vi "ROS_Publish.vi"() -> ()   [LabVIEW 2020]
uses:
  C:/Users/NI/Desktop/ROS/Release/ROSPublisherClass.dll
  Release/ROSPublisherClass.dll
panel:
  out "Numeric 2":i32
  out "Time 2":u32
  out "Time Array 2":u32[](array[numeric])
  out "Time Array":u32[](array[numeric])
  out "Time":u32
  out "Numeric":i32
  out "error out":errorcluster
  in  "stop":bool
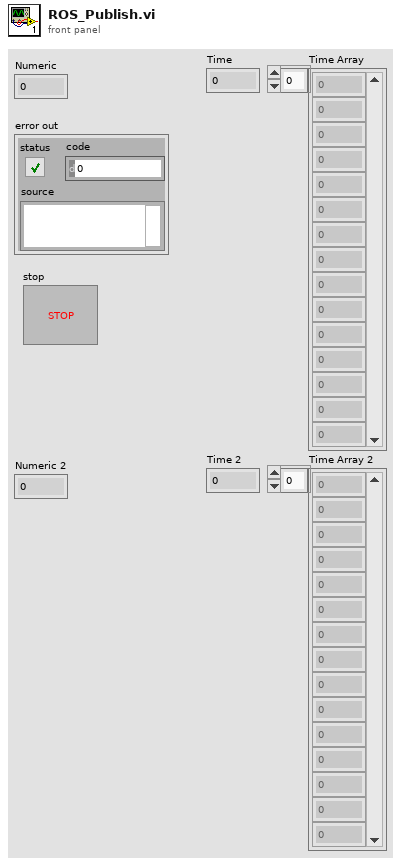
[diagram p1: front panel]
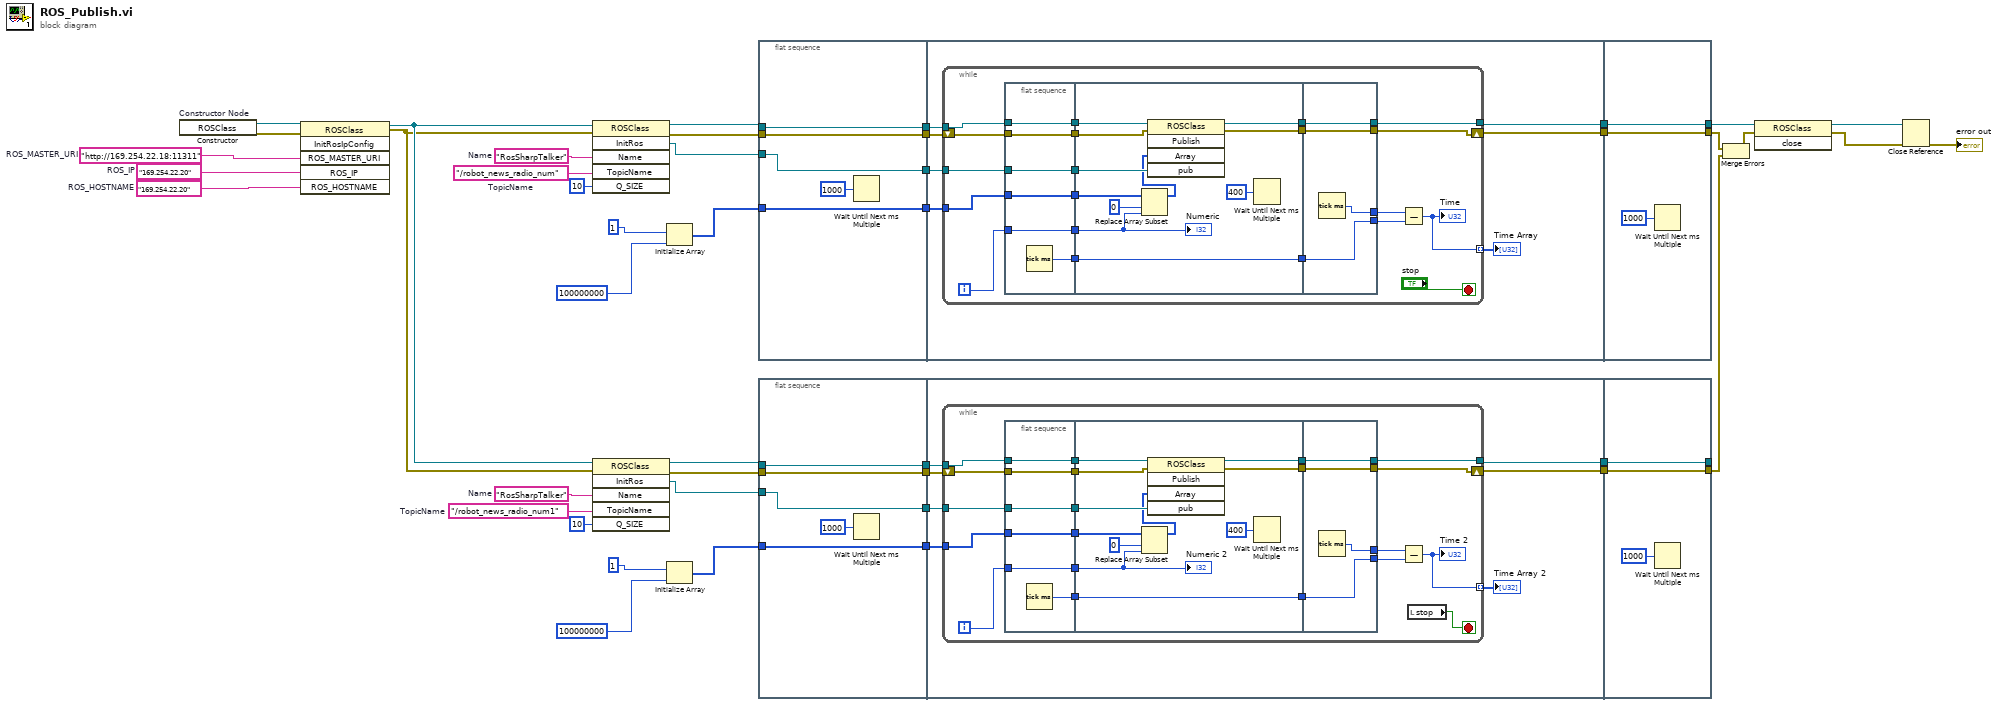
[diagram p0: block diagram]
diagram:
  w13 = "/robot_news_radio_num1"  # TopicName
  w12 = "RosSharpTalker"  # Name
  w22 = "/robot_news_radio_num"  # TopicName
  w23 = "RosSharpTalker"  # Name
  w24 = "169.254.22.20"  # ROS_HOSTNAME
  w26 = "http://169.254.22.18:11311"  # ROS_MASTER_URI
  w25 = "169.254.22.20"  # ROS_IP
  n1 = constructor on="Constructor Node" class="ROSClass"() -> (reference out=w41:refnum<k24>, error out=w30:errorcluster)  [unwired: 3 in, 1 out]
  n2 = invoke class="ROSClass" method="InitRosIpConfig"(reference=w41, error in=w30, "ROS_MASTER_URI"=w26, "ROS_IP"=w25, "ROS_HOSTNAME"=w24) -> (reference out=w5:refnum<k24>, error out=w4:errorcluster)  [unwired: 1 in, 4 out]
  n3 = invoke class="ROSClass" method="InitRos"(reference=w5, error in=w4, "Name"=w23, "TopicName"=w22, "Q_SIZE"=10) -> (reference out=w28:refnum<k24>, error out=w29:errorcluster, "InitRos"=w27:refnum<k24>)  [unwired: 1 in, 3 out]
  n4 = invoke class="ROSClass" method="InitRos"(reference=w5, error in=w4, "Name"=w12, "TopicName"=w13, "Q_SIZE"=10) -> (reference out=w10:refnum<k24>, error out=w9:errorcluster, "InitRos"=w11:refnum<k24>)  [unwired: 1 in, 3 out]
  n5 = Initialize Array(u8 1, 100000000 ("dimension size")) -> (w36:u8[])
  n6 = Initialize Array(u8 1, 100000000 ("dimension size")) -> (w8:u8[])
  n7 = flat-sequence {
    tunnel: w29 -> [w48]
    tunnel: w28 -> [w49]
    tunnel: [w49] -> w43
    tunnel: [w48] -> w42
    tunnel: w27 -> [w46]
    tunnel: [w46] -> w40
    tunnel: [w45] -> w37
    tunnel: w36 -> [w45]
    tunnel: w43 -> [w56]
    tunnel: w42 -> [w55]
    tunnel: w40 -> [w52]
    tunnel: w37 -> [w51]
    tunnel: [w54] -> w32
    tunnel: [w53] -> w31
    tunnel: [w99] -> w3
    tunnel: [w100] -> w44
    tunnel: w32 -> [w100]
    tunnel: w31 -> [w99]
    frame #0 {
      n8 = Wait Until Next ms Multiple(millisecond multiple=u32 1000) -> ()  [unwired: 1 out]
    }
    frame #1 {
      n9 = while {
        tunnel: w56 -> [w75]
        tunnel: [w74] -> w54
        shift-right: [w71] -> w53
        shift-left: w55 -> [w72]
        tunnel: w52 -> [w73]
        tunnel: w51 -> [w70]
        tunnel: [w57] -> w50 mode=indexing
        i -> [w69]
        stop <- "stop" stop-if-true
        n10 = flat-sequence {
          tunnel: w69 -> [w78]
          tunnel: w70 -> [w79]
          tunnel: w72 -> [w80]
          tunnel: w73 -> [w81]
          tunnel: w75 -> [w82]
          tunnel: [w82] -> w68
          tunnel: [w81] -> w67
          tunnel: [w80] -> w66
          tunnel: [w79] -> w65
          tunnel: [w78] -> w64
          tunnel: [w77] -> w58
          tunnel: w68 -> [w93]
          tunnel: w67 -> [w91]
          tunnel: w66 -> [w90]
          tunnel: w65 -> [w87]
          tunnel: w64 -> [w86]
          tunnel: [w92] -> w63
          tunnel: [w89] -> w62
          tunnel: [w83] -> w59
          tunnel: w58 -> [w83]
          tunnel: [w96] -> w71
          tunnel: [w97] -> w74
          tunnel: w63 -> [w97]
          tunnel: w62 -> [w96]
          tunnel: [w95] -> w61
          tunnel: [w94] -> w60
          tunnel: w59 -> [w94]
          frame #0 {
            n11 = Tick Count (ms)() -> (millisecond timer value=w77:u32)
          }
          frame #1 {
            n12 = Replace Array Subset(array=w87, new element=w86, index=0) -> (w84:u8[])
            n13 = invoke class="ROSClass" method="Publish"(reference=w93, error in=w90, "Array"=w84, "pub"=w91) -> (reference out=w92:refnum<k24>, error out=w89:errorcluster)  [unwired: 1 in, 3 out]
            n14 = Wait Until Next ms Multiple(millisecond multiple=u32 400) -> ()  [unwired: 1 out]
            "Numeric" <- w86
          }
          frame #2 {
            n15 = Tick Count (ms)() -> (millisecond timer value=w95:u32)
          }
        }
        n16 = Subtract(x=w61, y=w60) -> (x-y=w57:u32)
        "Time" <- w57
      }
      "Time Array" <- w50
    }
    frame #2 {
      n17 = Wait Until Next ms Multiple(millisecond multiple=u32 1000) -> ()  [unwired: 1 out]
    }
  }
  n18 = flat-sequence {
    tunnel: w9 -> [w104]
    tunnel: w10 -> [w105]
    tunnel: [w105] -> w20
    tunnel: [w104] -> w19
    tunnel: w11 -> [w102]
    tunnel: [w102] -> w18
    tunnel: [w101] -> w17
    tunnel: w8 -> [w101]
    tunnel: w20 -> [w112]
    tunnel: w19 -> [w111]
    tunnel: w18 -> [w108]
    tunnel: w17 -> [w107]
    tunnel: [w110] -> w16
    tunnel: [w109] -> w15
    tunnel: [w155] -> w1
    tunnel: [w156] -> _
    tunnel: w16 -> [w156]
    tunnel: w15 -> [w155]
    frame #0 {
      n19 = Wait Until Next ms Multiple(millisecond multiple=u32 1000) -> ()  [unwired: 1 out]
    }
    frame #1 {
      n20 = while {
        tunnel: w112 -> [w132]
        tunnel: [w131] -> w110
        shift-right: [w128] -> w109
        shift-left: w111 -> [w129]
        tunnel: w108 -> [w130]
        tunnel: w107 -> [w127]
        tunnel: [w114] -> w106 mode=indexing
        i -> [w126]
        stop <- w113 stop-if-true
        n21 = flat-sequence {
          tunnel: w126 -> [w134]
          tunnel: w127 -> [w135]
          tunnel: w129 -> [w136]
          tunnel: w130 -> [w137]
          tunnel: w132 -> [w138]
          tunnel: [w138] -> w125
          tunnel: [w137] -> w124
          tunnel: [w136] -> w123
          tunnel: [w135] -> w122
          tunnel: [w134] -> w121
          tunnel: [w133] -> w115
          tunnel: w125 -> [w149]
          tunnel: w124 -> [w147]
          tunnel: w123 -> [w146]
          tunnel: w122 -> [w143]
          tunnel: w121 -> [w142]
          tunnel: [w148] -> w120
          tunnel: [w145] -> w119
          tunnel: [w139] -> w116
          tunnel: w115 -> [w139]
          tunnel: [w152] -> w128
          tunnel: [w153] -> w131
          tunnel: w120 -> [w153]
          tunnel: w119 -> [w152]
          tunnel: [w151] -> w118
          tunnel: [w150] -> w117
          tunnel: w116 -> [w150]
          frame #0 {
            n22 = Tick Count (ms)() -> (millisecond timer value=w133:u32)
          }
          frame #1 {
            n23 = Replace Array Subset(array=w143, new element=w142, index=0) -> (w140:u8[])
            n24 = invoke class="ROSClass" method="Publish"(reference=w149, error in=w146, "Array"=w140, "pub"=w147) -> (reference out=w148:refnum<k24>, error out=w145:errorcluster)  [unwired: 1 in, 3 out]
            n25 = Wait Until Next ms Multiple(millisecond multiple=u32 400) -> ()  [unwired: 1 out]
            "Numeric 2" <- w142
          }
          frame #2 {
            n26 = Tick Count (ms)() -> (millisecond timer value=w151:u32)
          }
        }
        n27 = Subtract(x=w118, y=w117) -> (x-y=w114:u32)
        "Time 2" <- w114
        n28 = local read "stop"() -> (w113:bool)
      }
      "Time Array 2" <- w106
    }
    frame #2 {
      n29 = Wait Until Next ms Multiple(millisecond multiple=u32 1000) -> ()  [unwired: 1 out]
    }
  }
  n30 = Merge Errors(w3, w1) -> (w2:errorcluster)
  n31 = invoke class="ROSClass" method="close"(reference=w44, error in=w2) -> (reference out=w35:refnum<k24>, error out=w34:errorcluster)  [unwired: 1 in, 1 out]
  n32 = Close Reference(reference=w35, error in (no error)=w34) -> (error out=→"error out":errorcluster)
